vi "SW_Get_ROI_bounding_box.vi"(1 "Center of the ROI":T2, 2 "Radius of the ROI, pix":dbl format="%#_13g") -> (0 "Bounding box of the ROI, pix":T1)   [LabVIEW 2018]
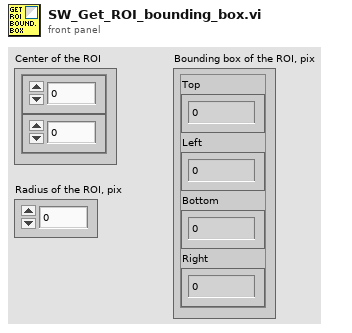
[diagram p1: front panel]
types:
  T1 = cluster{"Top":i32, "Left":i32, "Bottom":i32, "Right":i32}
  T2 = cluster{"Numeric Control":dbl, "Numeric Control":dbl}
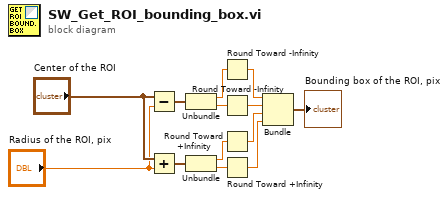
[diagram p0: block diagram]
diagram:
  n1 = Subtract(x="Center of the ROI", y="Radius of the ROI, pix") -> (x-y=w10:T2)
  n2 = Add(x="Center of the ROI", y="Radius of the ROI, pix") -> (x+y=w9:T2)
  n3 = Unbundle(w10) -> ("Numeric Control"=w8:dbl, "Numeric Control"=w7:dbl)
  n4 = Unbundle(w9) -> ("Numeric Control"=w6:dbl, "Numeric Control"=w5:dbl)
  n5 = Round Toward -Infinity(1:w8) -> (0:w4:dbl)
  n6 = Round Toward -Infinity(1:w7) -> (0:w3:dbl)
  n7 = Round Toward +Infinity(x=w6) -> (ceil(x): smallest int >= x=w2:dbl)
  n8 = Round Toward +Infinity(x=w5) -> (ceil(x): smallest int >= x=w1:dbl)
  n9 = Bundle(w4, w3, w2, w1) -> (→"Bounding box of the ROI, pix":cluster{dbl, dbl, dbl, dbl})  [unwired: 1 in]
